vi "Get Metadata.vi"(8 "error in (no error)":errorcluster, 11 "session id in":i32) -> (0 "error out":errorcluster, 2 "Metadata":string[][](table), 3 "session id out":i32)   [LabVIEW 2017, in "libonnx_wrapper.lvlib"]
uses:
  libonnx_wrapper.lvlib
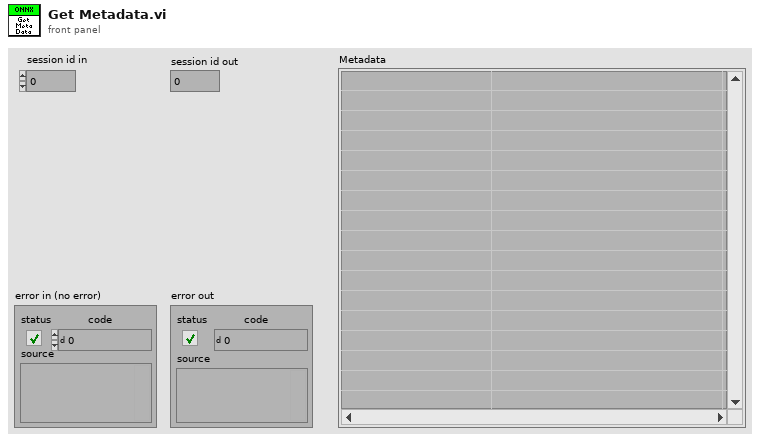
[diagram p1: front panel]
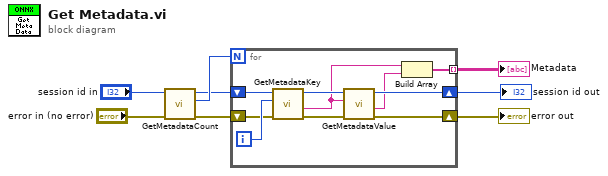
[diagram p0: block diagram]
diagram:
  n1 = call "GetMetadataCount.vi"("error in (no error)"="error in (no error)", "session id in"="session id in") -> ("error out"=w6:errorcluster, "MetadataCount"=w8:i32, "session id out"=w7:i32)  [unwired: 7 in]
  n2 = for {
    N: w8 -> [_]
    shift-right: [w13] -> w1
    shift-left: w7 -> [w18]
    shift-right: [w12] -> w3
    shift-left: w6 -> [w16]
    tunnel: [w9] -> w5 mode=indexing
    i -> [w17]
    n3 = call "GetMetadataKey.vi"("error in (no error)"=w16, "index"=w17, "session id in"=w18) -> ("error out"=w14:errorcluster, "MetadataKey"=w11:string, "session id out"=w15:i32)  [unwired: 5 in, 1 out]
    n4 = call "GetMetadataValue.vi"("error in (no error)"=w14, "key"=w11, "session id in"=w15) -> ("error out"=w12:errorcluster, "MetadataKey"=w10:string, "session id out"=w13:i32)  [unwired: 5 in, 1 out]
    n5 = Build Array(w11, w10) -> (w9:string[])
  }
  "Metadata" <- w5
  "error out" <- w3
  "session id out" <- w1
